vi "ErrorLatch.vi"(1 "Trigger":bool) -> (0 "Latched":bool)   [LabVIEW 2019]
doc: "This VI will latch an error flag until cleared or suppressed (overriden). This VI is designed for integration with global variables to read the error clear and override signals."
uses:
  dsdata.vi
  dscommands.vi
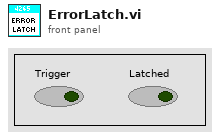
[diagram p1: front panel]
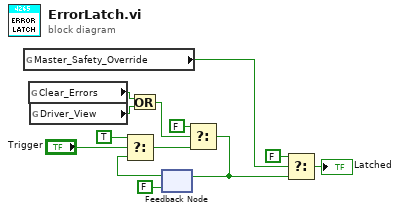
[diagram p0: block diagram]
diagram:
  n1 = global read "dsdata.vi" "Master_Safety_Override"() -> (w4:bool)
  n2 = global read "dsdata.vi" "Clear_Errors"() -> (w3:bool)
  n3 = global read "dscommands.vi" "Driver_View"() -> (w2:bool)
  n4 = Or(x=w3, y=w2) -> (x .or. y?=w1:bool)
  n5 = feedback #1(FALSE) -> (w12:bool)
  n6 = Select(t=TRUE, s="Trigger", f=w12) -> (s? t:f=w9:bool)
  n7 = Select(t=FALSE, s=w1, f=w9) -> (s? t:f=w7:bool)
  n8 = feedback-in #1(w7) -> ()
  n9 = Select(t=FALSE, s=w4, f=w7) -> (s? t:f=→"Latched":bool)
